vi "Format Image Description Row.vi"(7 "Column Count":i32, 8 "error in (no error)":errorcluster {"code" format="Error %.0f"}, 10 "Image Structure":string, 11 "Description":string) -> (0 "error out":errorcluster {"code" format="Error %.0f"}, 2 "Table Row Text":string)   [LabVIEW 2023, in "VIDoc Printer - Confluence.lvlib" / "VIDoc Printer - Confluence.lvclass"]
uses:
  VIDoc Printer - Confluence.lvclass
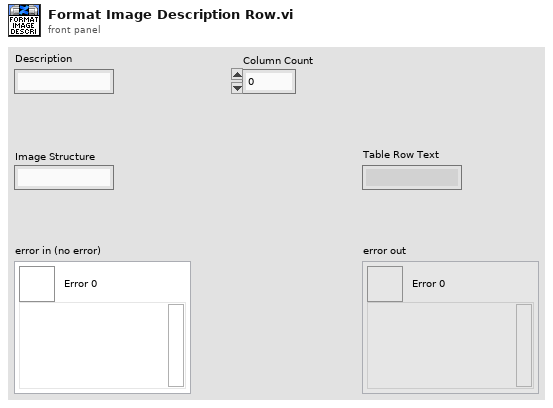
[diagram p1: front panel]
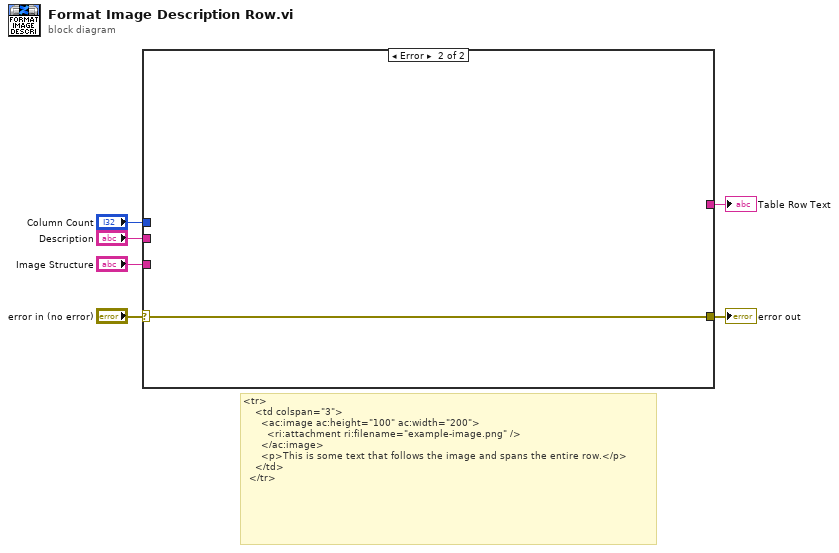
[diagram p0: block diagram]
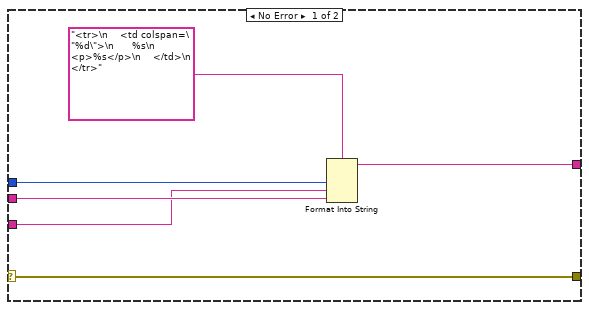
[diagram p2: hidden frame]
diagram:
  # "<tr>\n    <td colspan=\"3\">\n      <ac:image ac:height=\"100\" ac:width=\"200\">\n        <ri:attachment ri:filename=\"example-image.png\" />\n      </ac:image>\n      <p>This is some text that follows the image and spans the entire row.</p>\n    </td>\n  </tr>"
  n1 = case shown="Error" "error in (no error)" {
    selector: "error in (no error)" -> [w7 w13]
    tunnel: [w7 w13] -> w5
    tunnel: "Column Count" -> [w11 _]
    tunnel: "Description" -> [w10 _]
    tunnel: [w9 _] -> w2
    tunnel: "Image Structure" -> [w8 _]
    frame No Error {
      n2 = Format Into String(format string="<tr>\n    <td colspan=\"%d\">\n      %s\n      <p>%s</p>\n    </td>\n  </tr>", w11, w8, w10) -> (resulting string=w9:string)  [unwired: 2 in, 1 out]
    }
    frame Error {
    }
  }
  "error out" <- w5
  "Table Row Text" <- w2
